vi "GoToBallKeeperSkillVSS.vi"(8 "error in (no error)":errorcluster, 9 "Robot in":refnum<class "Robot.lvclass">, 10 "Game in":refnum<class "Game.lvclass">, 11 "GoToBallKeeperSkillVSS in":refnum<class "GoToBallKeeperSkillVSS.lvclass">) -> (0 "error out":errorcluster, 1 "Robot out":refnum<class "Robot.lvclass">, 3 "GoToBallKeeperSkillVSS out":refnum<class "GoToBallKeeperSkillVSS.lvclass">)   [LabVIEW 2023, in "GoToBallKeeperSkillVSS.lvclass"]
uses:
  GoToBallKeeperSkillVSS.lvclass
  Robot_class/Robot.lvclass
  Game_class/Game.lvclass
  Game_class/Game.lvclass/Game.ctl
  Object_class/Object.lvclass/Object.ctl
  Robot_class/Robot.lvclass/Robot.ctl
  Game_class/Read BallRef.vi
  Game_class/Read FieldRef.vi
  Object_class/Read x.vi
  Object_class/Read y.vi
  Robot_class/Write dest_x.vi
  Robot_class/Write dest_y.vi
  Robot_class/Write dest_orientation.vi
  Ball_class/Ball.lvclass
  Field_class/Field.lvclass
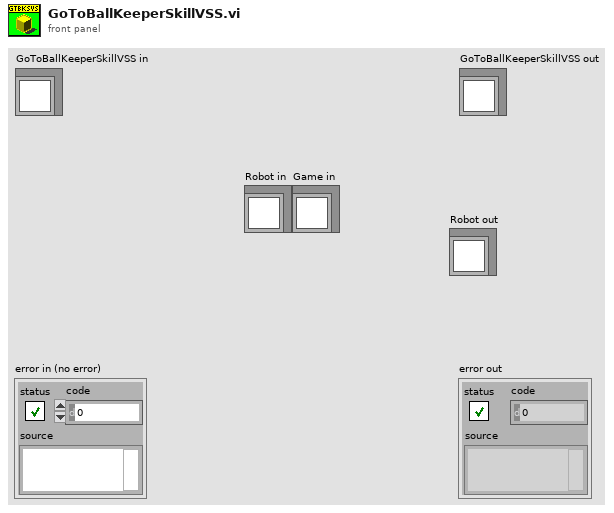
[diagram p1: front panel]
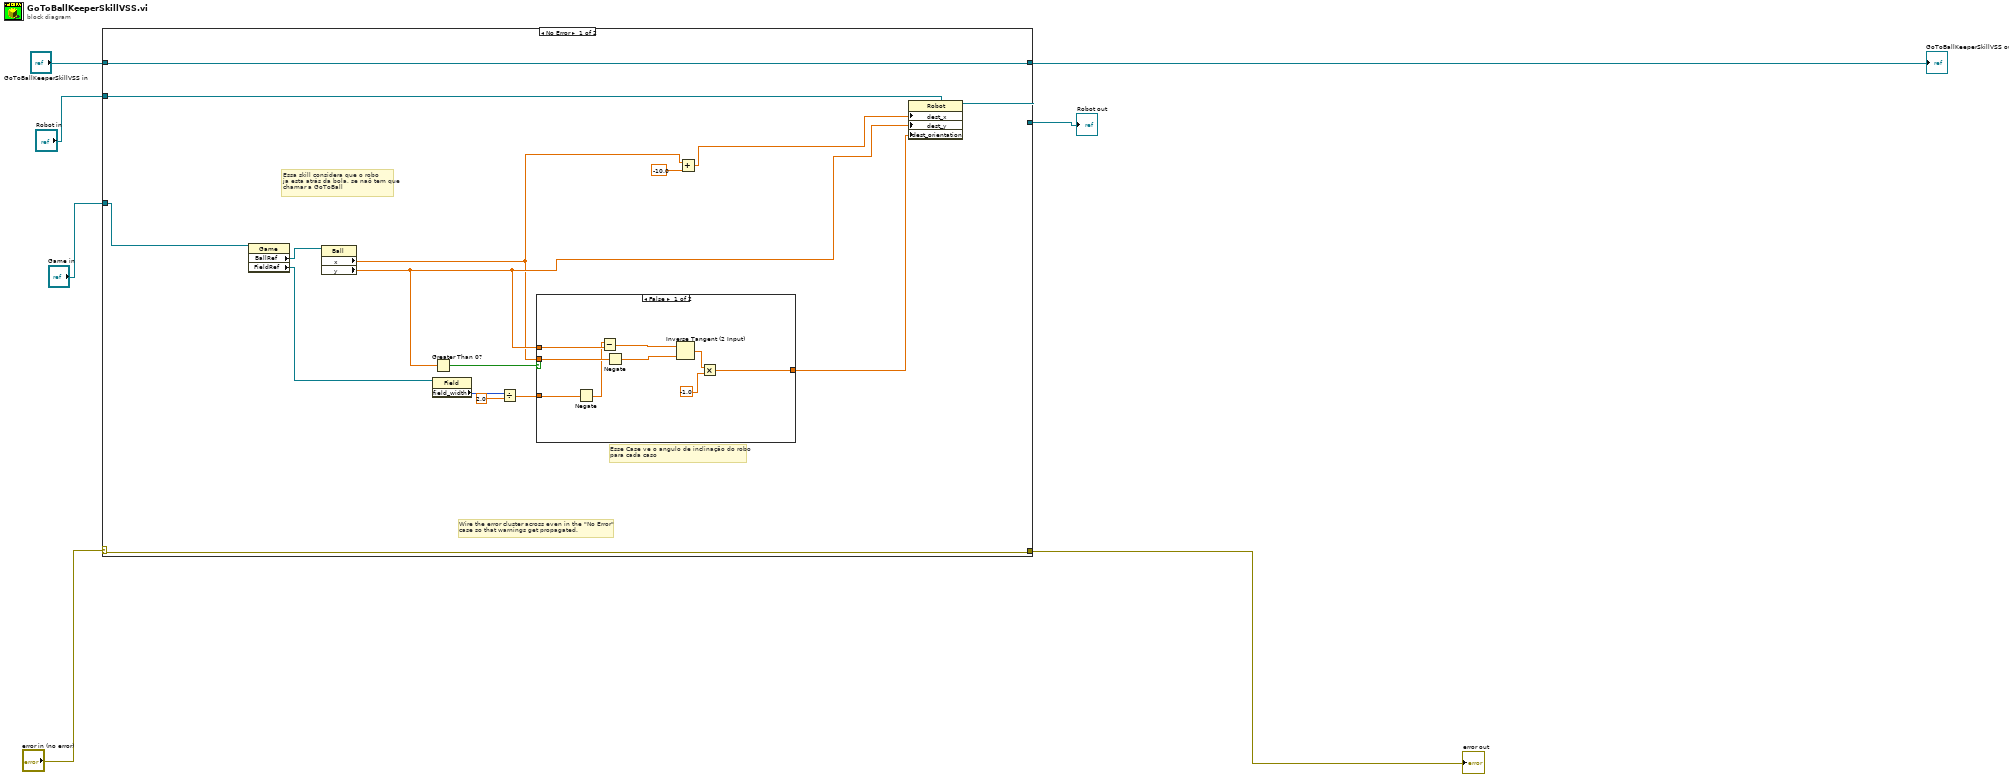
[diagram p0: block diagram]
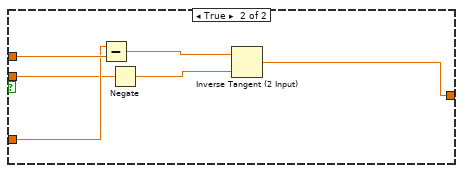
[diagram p2: hidden frame]
diagram:
  n1 = case shown="No Error" "error in (no error)" {
    selector: "error in (no error)" -> [w22 w41]
    tunnel: [w22 w41] -> w6
    tunnel: [w23 w40] -> w4
    tunnel: "GoToBallKeeperSkillVSS in" -> [w23 w40]
    tunnel: "Robot in" -> [w20 w39]
    tunnel: [w21 w39] -> w2
    tunnel: "Game in" -> [w17 _]
    frame No Error {
      # "Esse Case ve o angulo de inclinação do robo\npara cada caso"
      # "Essa skill considera que o robo \nja esta atrás da bola, se naõ tem que\nchamar a GoToBall"
      # "Wire the error cluster across even in the \"No Error\"\ncase so that warnings get propagated."
      n2 = property class="Game"(reference=w17) -> ("BallRef"=w19:refnum<class "Ball.lvclass">, "FieldRef"=w15:refnum<class "Field.lvclass">)  [unwired: 1 in, 2 out]
      n3 = property class="Ball"(reference=w19) -> ("x"=w9:dbl, "y"=w11:dbl)  [unwired: 1 in, 2 out]
      n4 = property class="Field"(reference=w15) -> ("field_width"=w13:i32)  [unwired: 1 in, 2 out]
      n5 = Greater Than 0?(x=w11) -> (x > 0?=w14:bool)
      n6 = Divide(x=w13, y=2.0) -> (x/y=w10:dbl)
      n7 = case shown="False" w14 {
        tunnel: w11 -> [w30 w38]
        tunnel: w10 -> [w25 w37]
        tunnel: w9 -> [w29 w35]
        tunnel: [w26 w33] -> w8
        frame False {
          n8 = Negate(x=w25) -> (-x=w24:dbl)
          n9 = Subtract(x=w24, y=w30) -> (x-y=w32:dbl)
          n10 = Negate(x=w29) -> (-x=w31:dbl)
          n11 = Inverse Tangent (2 Input)(1:w31, 2:w32) -> (0:w27:dbl)
          n12 = Multiply(x=w27, y=-1.0) -> (x*y=w26:dbl)
        }
        frame True {
          n13 = Subtract(x=w37, y=w38) -> (x-y=w36:dbl)
          n14 = Negate(x=w35) -> (-x=w34:dbl)
          n15 = Inverse Tangent (2 Input)(1:w34, 2:w36) -> (0:w33:dbl)
        }
      }
      n16 = Add(x=w9, y=-10.0) -> (x+y=w16:dbl)
      n17 = property class="Robot"(reference=w20, "dest_x"=w16, "dest_y"=w11, "dest_orientation"=w8) -> (reference out=w21:refnum<class "Robot.lvclass">)  [unwired: 1 in, 1 out]
    }
    frame Error {
    }
  }
  "error out" <- w6
  "GoToBallKeeperSkillVSS out" <- w4
  "Robot out" <- w2
